vi "numer timeser inator.vi"() -> ()   [LabVIEW 2021]
uses:
  <vilib>/numeric/Random Number (Range) I64.vi
  <vilib>/numeric/sub_Random U32.vi
panel:
  out "Array 4":string[](array[string])
  out "Array 3":dbl[](array[numeric])
  out "XY Graph":cluster{i32[], dbl[]}(graph)
  out "Array 2":dbl[](array[numeric])
  out "Array":dbl[](array[numeric])
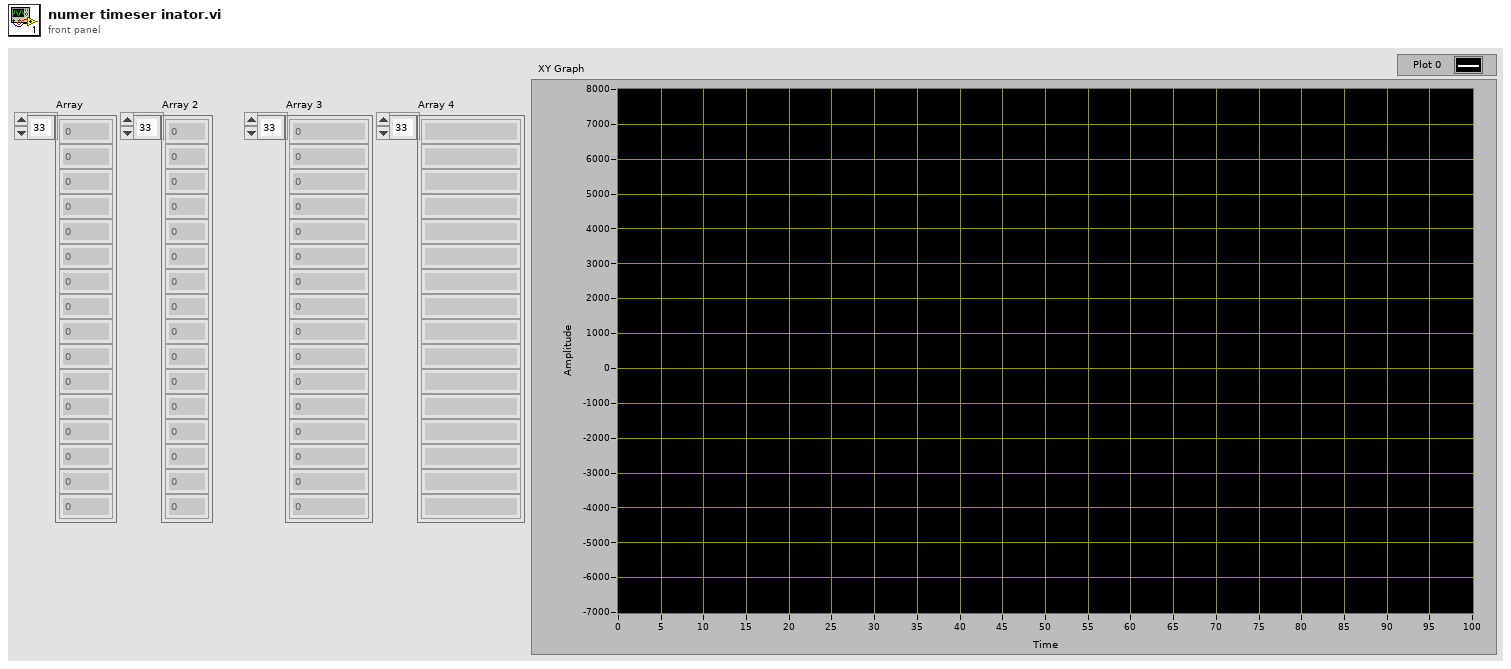
[diagram p1: front panel]
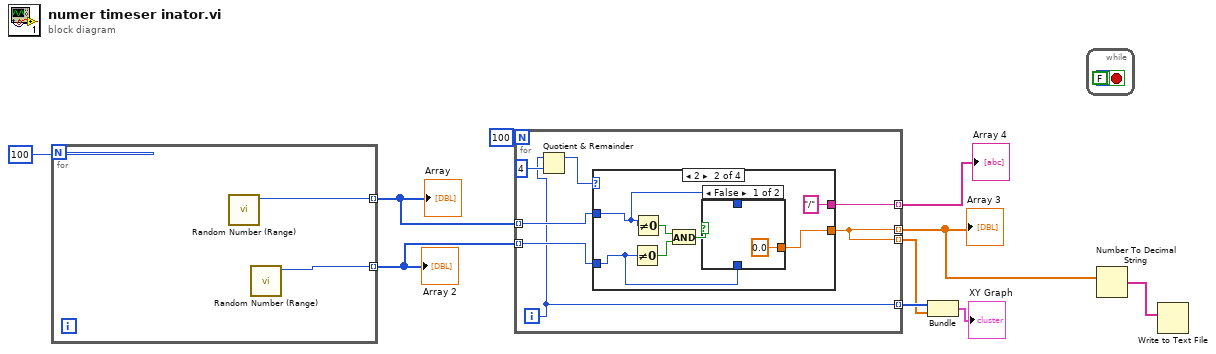
[diagram p0: block diagram]
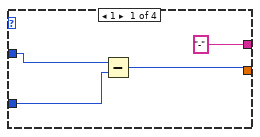
[diagram p2: hidden frame]
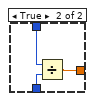
[diagram p3: hidden frame]
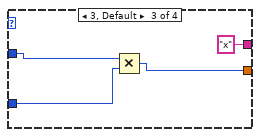
[diagram p4: hidden frame]
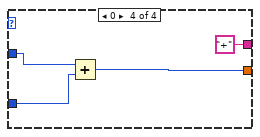
[diagram p5: hidden frame]
diagram:
  n1 = for {
    N: 100 -> [_]
    tunnel: [w12] -> w8 mode=indexing
    tunnel: [w11] -> w7 mode=indexing
    n2 = call-poly <vilib>:"Random Number (Range).vi"() -> ("number"=w12:i64)  [unwired: 11 in]
    n3 = call-poly <vilib>:"Random Number (Range).vi"() -> ("number"=w11:i64)  [unwired: 11 in]
  }
  "Array" <- w8
  "Array 2" <- w7
  n4 = for {
    N: 100 -> [_]
    tunnel: w8 -> [w18] mode=indexing
    tunnel: w7 -> [w17] mode=indexing
    tunnel: [w14] -> w2 mode=indexing
    tunnel: [w15] -> w6 mode=indexing
    tunnel: [w14] -> w5 mode=indexing
    tunnel: [w13] -> w3 mode=indexing
    i -> [w15]
    n5 = Quotient & Remainder(x=w15, y=4) -> (x-y*floor(x/y)=w16:i32)  [unwired: 1 out]
    n6 = case shown="2" w16 {
      tunnel: w18 -> [w23 w25 w38 w42]
      tunnel: w17 -> [w22 w24 w37 w41]
      tunnel: [w21 w29 w36 w40] -> w14
      tunnel: ["-" "/" "x" "+"] -> w13
      frame 1 {
        n7 = Subtract(x=w23, y=w22) -> (x-y=w21:i64)
      }
      frame 2 {
        n8 = Not Equal To 0?(x=w24) -> (x != 0?=w27:bool)
        n9 = Not Equal To 0?(x=w25) -> (x != 0?=w28:bool)
        n10 = And(x=w28, y=w27) -> (x .and. y?=w26:bool)
        n11 = case shown="False" w26 {
          tunnel: [0.0 w34] -> w29
          tunnel: w25 -> [_ w33]
          tunnel: w24 -> [_ w32]
          frame False {
          }
          frame True {
            n12 = Divide(x=w33, y=w32) -> (x/y=w34:dbl)
          }
        }
      }
      frame 3, Default {
        n13 = Multiply(x=w38, y=w37) -> (x*y=w36:i64)
      }
      frame 0 {
        n14 = Add(x=w42, y=w41) -> (x+y=w40:i64)
      }
    }
  }
  "Array 3" <- w2
  "Array 4" <- w3
  n15 = Bundle(w6, w5) -> (→"XY Graph":cluster{i32[], dbl[]})  [unwired: 1 in]
  n16 = while {
    stop <- FALSE stop-if-true
  }
  n17 = Number To Decimal String(number=w2) -> (decimal integer string=w1:string[])  [unwired: 1 in]
  n18 = Write to Text File(text=w1) -> ()  [unwired: 3 in, 3 out]
